vi "Apply Selected Labels to Control.vi"(8 "error in (no error)":errorcluster, 10 "Alternate Text Select (0)":i32, 11 "Waveform Graph in":refnum<class "Waveform Chart.lvclass">) -> (0 "error out":errorcluster, 3 "Waveform Graph out":refnum<class "Waveform Chart.lvclass">)   [LabVIEW 2017, in "Localization.lvlib" / "Waveform Chart.lvclass"]
doc: "Use the information in the class to apply the selected alternate text from the Additional Labels to the control.\n\nChoose Movement Consulting, LLC"
uses:
  Waveform Chart.lvclass
  C:/Apps/CMC/OpenSource/Localization/Control Info/Control Info.lvclass
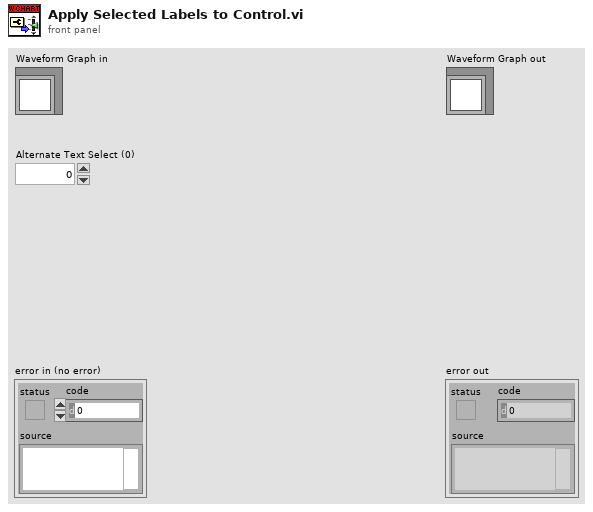
[diagram p1: front panel]
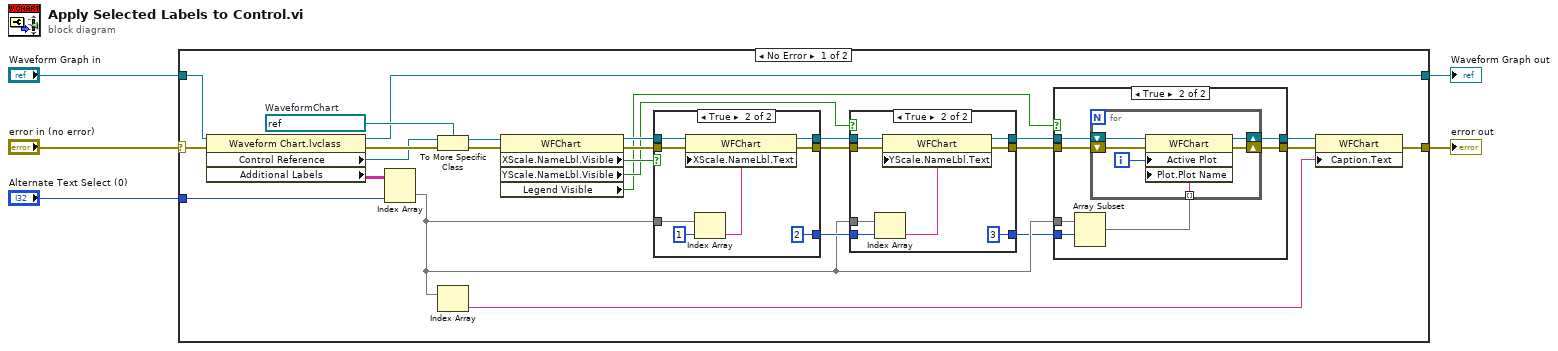
[diagram p0: block diagram]
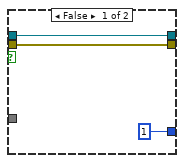
[diagram p4: hidden frame]
diagram:
  n1 = case shown="No Error" "error in (no error)" {
    selector: "error in (no error)" -> [w26 w70]
    tunnel: "Waveform Graph in" -> [w25 w69]
    tunnel: [w21 w70] -> w2
    tunnel: [w22 w69] -> w1
    tunnel: "Alternate Text Select (0)" -> [w23 _]
    frame No Error {
      w31 = refnum<vi> refnum  # WaveformChart
      n2 = property class="Waveform Chart.lvclass"(reference=w25, error in=w26) -> (reference out=w22:refnum<class "Waveform Chart.lvclass">, error out=w28:errorcluster, "Control Reference"=w27:refnum<vi>, "Additional Labels"=w24:string[][])
      n3 = Index Array(array=w24, index (col)=w23) -> (element=w12:string[])  [unwired: 1 in]
      n4 = To More Specific Class(target class=w31, reference=w27, error in=w28) -> (specific class reference=w30:refnum<vi>, error out=w29:errorcluster)
      n5 = Index Array(array=w12) -> (element=w20:string)  [unwired: 1 in]
      n6 = property class="WFChart"(reference=w30, error in=w29) -> (reference out=w19:refnum<vi>, error out=w18:errorcluster, "XScale.NameLbl.Visible"=w17:bool, "YScale.NameLbl.Visible"=w13:bool, "Legend Visible"=w6:bool)
      n7 = case shown="True" w17 {
        tunnel: w19 -> [w60 w68]
        tunnel: w18 -> [w59 w67]
        tunnel: [w60 w66] -> w16
        tunnel: [w59 w65] -> w15
        tunnel: w12 -> [_ w64]
        tunnel: [1 ("index") 2 ("index")] -> w14
        frame False {
        }
        frame True {
          n8 = Index Array(array=w64, index=1) -> (element=w62:string)
          n9 = property class="WFChart"(reference=w68, error in=w67, "XScale.NameLbl.Text"=w62) -> (reference out=w66:refnum<vi>, error out=w65:errorcluster)
        }
      }
      n10 = case shown="True" w13 {
        tunnel: w16 -> [w49 w57]
        tunnel: w15 -> [w48 w56]
        tunnel: w12 -> [_ w55]
        tunnel: w14 -> [w47 w54]
        tunnel: [w49 w52] -> w11
        tunnel: [w48 w51] -> w10
        tunnel: [w47 3 ("index")] -> w9
        frame False {
        }
        frame True {
          n11 = Index Array(array=w55, index=w54) -> (element=w53:string)
          n12 = property class="WFChart"(reference=w57, error in=w56, "YScale.NameLbl.Text"=w53) -> (reference out=w52:refnum<vi>, error out=w51:errorcluster)
        }
      }
      n13 = case shown="True" w6 {
        tunnel: w11 -> [w33 w40]
        tunnel: w10 -> [w32 w39]
        tunnel: w12 -> [_ w38]
        tunnel: w9 -> [_ w37]
        tunnel: [w33 w35] -> w8
        tunnel: [w32 w34] -> w7
        frame False {
        }
        frame True {
          n14 = Array Subset(array=w38, index=w37) -> (w36:string[])  [unwired: 1 in]
          n15 = for {
            tunnel: w36 -> [w43] mode=indexing
            shift-right: [w42] -> w35
            shift-left: w40 -> [w46]
            shift-right: [w41] -> w34
            shift-left: w39 -> [w45]
            i -> [w44]
            n16 = property class="WFChart"(reference=w46, error in=w45, "Active Plot"=w44, "Plot.Plot Name"=w43) -> (reference out=w42:refnum<vi>, error out=w41:errorcluster)
          }
        }
      }
      n17 = property class="WFChart"(reference=w8, error in=w7, "Caption.Text"=w20) -> (error out=w21:errorcluster)  [unwired: 1 out]
    }
    frame Error {
    }
  }
  "error out" <- w2
  "Waveform Graph out" <- w1
